vi "Actor Receive.vi"(11 "Dev Actor in":refnum<class "Dev Actor.lvclass">) -> (0 "error out":errorcluster, 2 "Msg":refnum<class "Msg Strategy.lvclass">, 3 "Dev Actor out":refnum<class "Dev Actor.lvclass">)   [LabVIEW 2021, in "Dev Actor.lvlib" / "Dev Actor.lvclass"]
uses:
  Dev Actor.lvclass
  src/LVCAM/LVCAM/Msg Strategy/Msg Strategy.lvclass
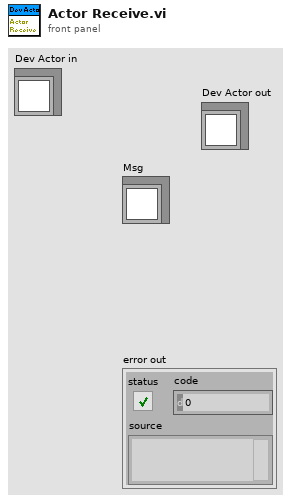
[diagram p1: front panel]
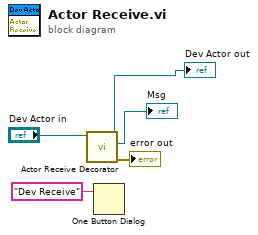
[diagram p0: block diagram]
diagram:
  n1 = call "Actor Receive Decorator.vi"("Dev Actor in"="Dev Actor in") -> ("error out"=→"error out":errorcluster, "Msg"=→"Msg":refnum<class "Msg Strategy.lvclass">, "Dev Actor out"=→"Dev Actor out":refnum<class "Dev Actor.lvclass">)  [unwired: 8 in]
  n2 = One Button Dialog(message="Dev Receive") -> ()  [unwired: 1 in, 1 out]
